vi "SMU Channel Output Control.vi"(0 "Semiconductor Module Context":T1, 2 "output enabled?":bool=TRUE caption="output enabled", 5 "Pins":string[](array[string]), 11 "error in (no error)":errorcluster) -> (15 "error Out":errorcluster)   [LabVIEW 2013]
uses:
  <vilib>/NI_TestStand_SemiconductorModule/NI_TestStand_Semiconductor_Module.lvlibp/PinMap/General/SemiconductorModuleContext.ctl
  <vilib>/NI_TestStand_SemiconductorModule/NI_TestStand_Semiconductor_Module.lvlibp/PinMap/DC Power/PinsToNIDCPowerSessions.vi
  <vilib>/NI_TestStand_SemiconductorModule/NI_TestStand_Semiconductor_Module.lvlibp
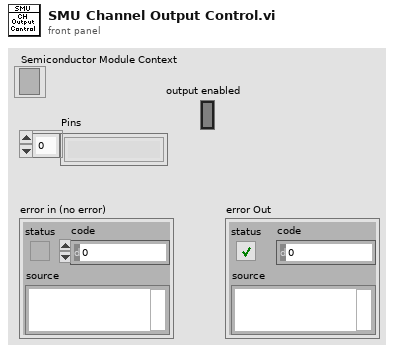
[diagram p1: front panel]
types:
  T1 = typedef "NI_TestStand_Semiconductor_Module.lvlibp/SemiconductorModuleContext.ctl" = refnum<k7>
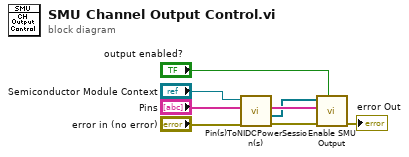
[diagram p0: block diagram]
diagram:
  n1 = call-poly <vilib>:"Pin(s)ToNIDCPowerSession(s).vi"("error in (no error)"="error in (no error)", "Pins"="Pins", "Semiconductor Module Context"="Semiconductor Module Context") -> ("error out"=w5:errorcluster, "Instrument Sessions"=w3:refnum<k15>[], "Channel Lists"=w4:string[])  [unwired: 4 in, 2 out]
  n2 = call "Enable SMU Output.vi"("output enabled"="output enabled?", "error in (no error)"=w5, "Channel Lists"=w4, "Instrument Sessions In"=w3) -> ("error Out"=→"error Out":errorcluster)  [unwired: 6 in, 1 out]
